vi "Z complex to magnitude phase.vi"(6 "Angle unit":enum16{"Radians", "Degrees"}(ring), 8 "Error In":errorcluster, 9 "Z (cplx)":T2 {"Z" format="%#_4g"}) -> (0 "Error Out":errorcluster, 1 "arg Z":T1, 2 "|Z|":T1)   [LabVIEW 2016]
uses:
  Trace (cplx).ctl
  Trace (dbl).ctl
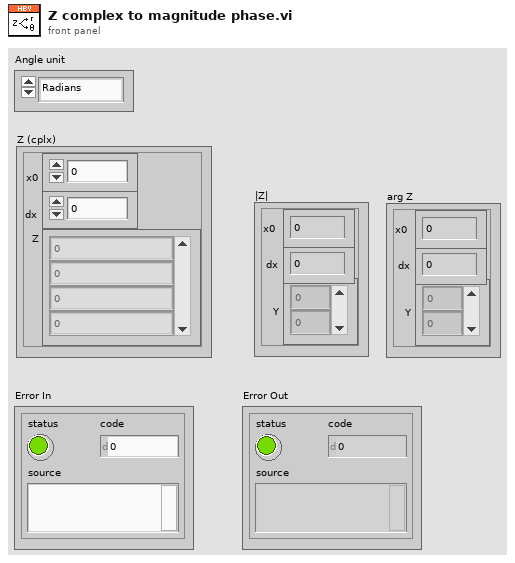
[diagram p1: front panel]
types:
  T1 = typedef "Trace (dbl).ctl" = cluster{"x0 ":dbl, "dx":dbl, "Y":dbl[]}
  T2 = typedef "Trace (cplx).ctl" = cluster{"x0":dbl, "dx":dbl, "Z":cdb[]}
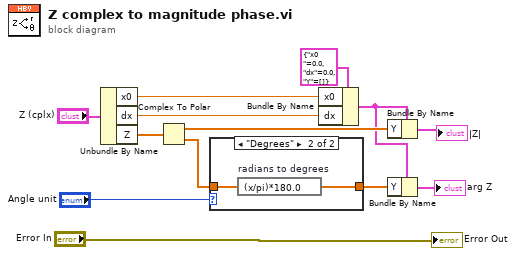
[diagram p0: block diagram]
diagram:
  n1 = Unbundle By Name("Z (cplx)") -> ("x0"=w7:dbl, "dx"=w6:dbl, "Z"=w3:cdb[])
  n2 = Complex To Polar(r * e^(i*theta)=w3) -> (r=w11:dbl[], theta=w10:dbl[])
  n3 = case shown="\"Degrees\"" "Angle unit" {
    tunnel: [w14 w16] -> w13
    tunnel: w10 -> [w14 w15]
    frame "Radians", Default {
    }
    frame "Degrees" {
      n4 = expression code="(x/pi)*180.0" "radians to degrees"(w15) -> (w16:dbl[])
    }
  }
  n5 = Bundle By Name(cluster=T1 {"x0 "=0.0, "dx"=0.0, "Y"=[]} ("Spectrum"), "x0"=w7, "dx"=w6) -> (w4:T1)
  n6 = Bundle By Name(cluster=w4, "Y"=w11) -> (→"|Z|":T1)
  n7 = Bundle By Name(cluster=w4, "Y"=w13) -> (→"arg Z":T1)
  "Error Out" <- "Error In"
